vi "Move Forward.vi"(8 "error in (no error)":errorcluster, 11 "Stage Controller in":refnum<class "Stage Controller.lvclass">) -> (0 "error out":errorcluster, 3 "Stage Controller out":refnum<class "Stage Controller.lvclass">)   [LabVIEW 2018, in "Stage Controller.lvlib" / "Stage Controller.lvclass"]
uses:
  Stage Controller.lvclass
  Stage Controller.lvclass/Stage Controller.ctl
  Ti2/ti2lv/ti2lv.lvlib
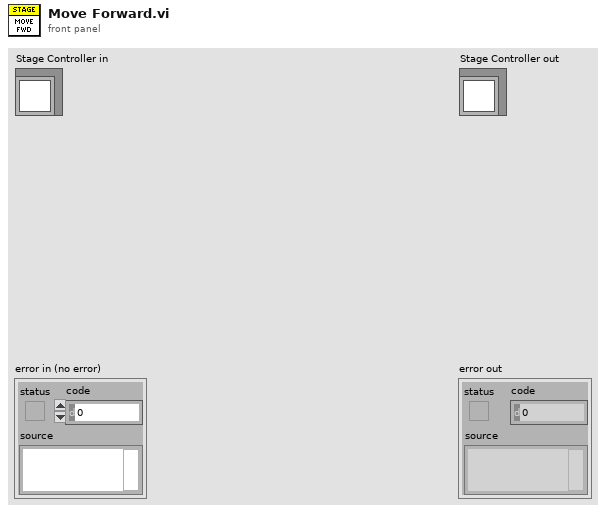
[diagram p1: front panel]
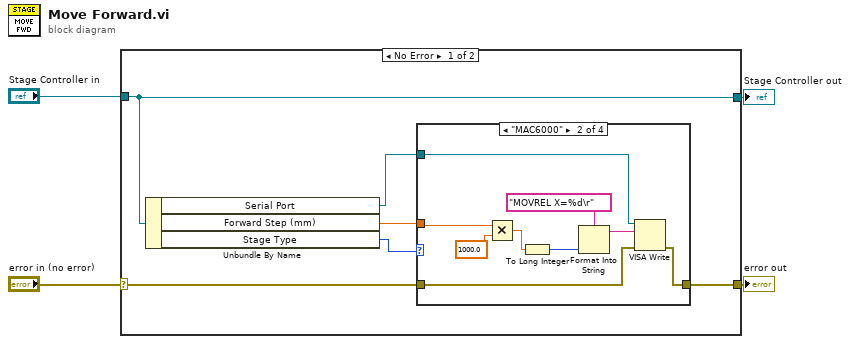
[diagram p0: block diagram]
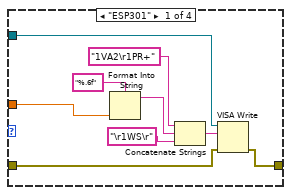
[diagram p2: hidden frame]
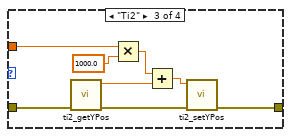
[diagram p3: hidden frame]
diagram:
  n1 = case shown="No Error" "error in (no error)" {
    selector: "error in (no error)" -> [w8 w39]
    tunnel: [w5 w39] -> w3
    tunnel: [w10 w38] -> w1
    tunnel: "Stage Controller in" -> [w10 w38]
    frame No Error {
      n2 = Unbundle By Name(w10) -> ("Serial Port"=w7:refnum<visa-resource-name>, "Forward Step (mm)"=w9:dbl, "Stage Type"=w6:enum16{"Disabled", "ESP301", "Ti2", "MAC6000"})
      n3 = case shown="\"MAC6000\"" w6 {
        tunnel: w9 -> [w12 w20 w35 _]
        tunnel: [w14 w23 w33 w37] -> w5
        tunnel: w8 -> [w13 w22 w32 w37]
        tunnel: w7 -> [w11 w21 _ _]
        frame "ESP301" {
          n4 = Format Into String(format string="%.6f", w12) -> (resulting string=w18:string)  [unwired: 2 in, 1 out]
          n5 = Concatenate Strings("1VA2\r1PR+" ("write buffer"), w18, "\r1WS\r" ("write buffer")) -> (w19:string)
          n6 = VISA Write(VISA resource name=w11, write buffer=w19, error in (no error)=w13) -> (error out=w14:errorcluster)  [unwired: 2 out]
        }
        frame "MAC6000" {
          n7 = Multiply(x=w20, y=1000.0) -> (x*y=w24:dbl)
          n8 = To Long Integer(number=w24) -> (32bit integer=w25:i32)
          n9 = Format Into String(format string="MOVREL X=%d\r", w25) -> (resulting string=w27:string)  [unwired: 2 in, 1 out]
          n10 = VISA Write(VISA resource name=w21, write buffer=w27, error in (no error)=w22) -> (error out=w23:errorcluster)  [unwired: 2 out]
        }
        frame "Ti2" {
          n11 = call "ti2_getYPos.vi"("error in (no error)"=w32) -> ("error out"=w31:errorcluster, "y Position (um)"=w29:dbl)  [unwired: 9 in]
          n12 = Multiply(x=w35, y=1000.0) -> (x*y=w36:dbl)
          n13 = Add(x=w36, y=w29) -> (x+y=w30:dbl)
          n14 = call "ti2_setYPos.vi"("error in (no error)"=w31, "y Position (um)"=w30) -> ("error out"=w33:errorcluster)  [unwired: 9 in]
        }
        frame "Disabled", Default {
        }
      }
    }
    frame Error {
    }
  }
  "error out" <- w3
  "Stage Controller out" <- w1
